vi "Untitled 2 (pub).vi"() -> (0 "error out":errorcluster, 2 "Array 3":dbl[](array[numeric]), 3 "Message":string)   [LabVIEW 2016]
uses:
  builds/UnicornMain/UnicornRIO1/ROS for LabVIEW/home/lvuser/natinst/bin/user.lib/ROS for LabVIEW Software/ROS/Code/SubVIs/_ROSControl.ctl
  builds/UnicornMain/UnicornRIO1/ROS for LabVIEW/home/lvuser/natinst/bin/user.lib/ROS for LabVIEW Software/ROS/Code/SubVIs/_ROSDirection.ctl
  builds/UnicornMain/UnicornRIO1/ROS for LabVIEW/home/lvuser/natinst/bin/user.lib/ROS for LabVIEW Software/ROS/Code/Console/Servers/ServerSubs/TopicDef.ctl
  GlobalVI.vi
  Global 2.vi
  builds/UnicornMain/UnicornRIO1/ROS for LabVIEW/home/lvuser/natinst/bin/user.lib/ROS for LabVIEW Software/ROS/Code/_ROSDefinition.vi
panel:
  out "JSON string 2":string
  out "ROS out":T1={"topic port"=0, "Node"="", "topic"="", "type"="", "node port"=0, "error "={"status"=FALSE, "code"=0, "source"=""}, "Direction"=enum."Node", "Update (ms)"=1, "FIFO size"=1}
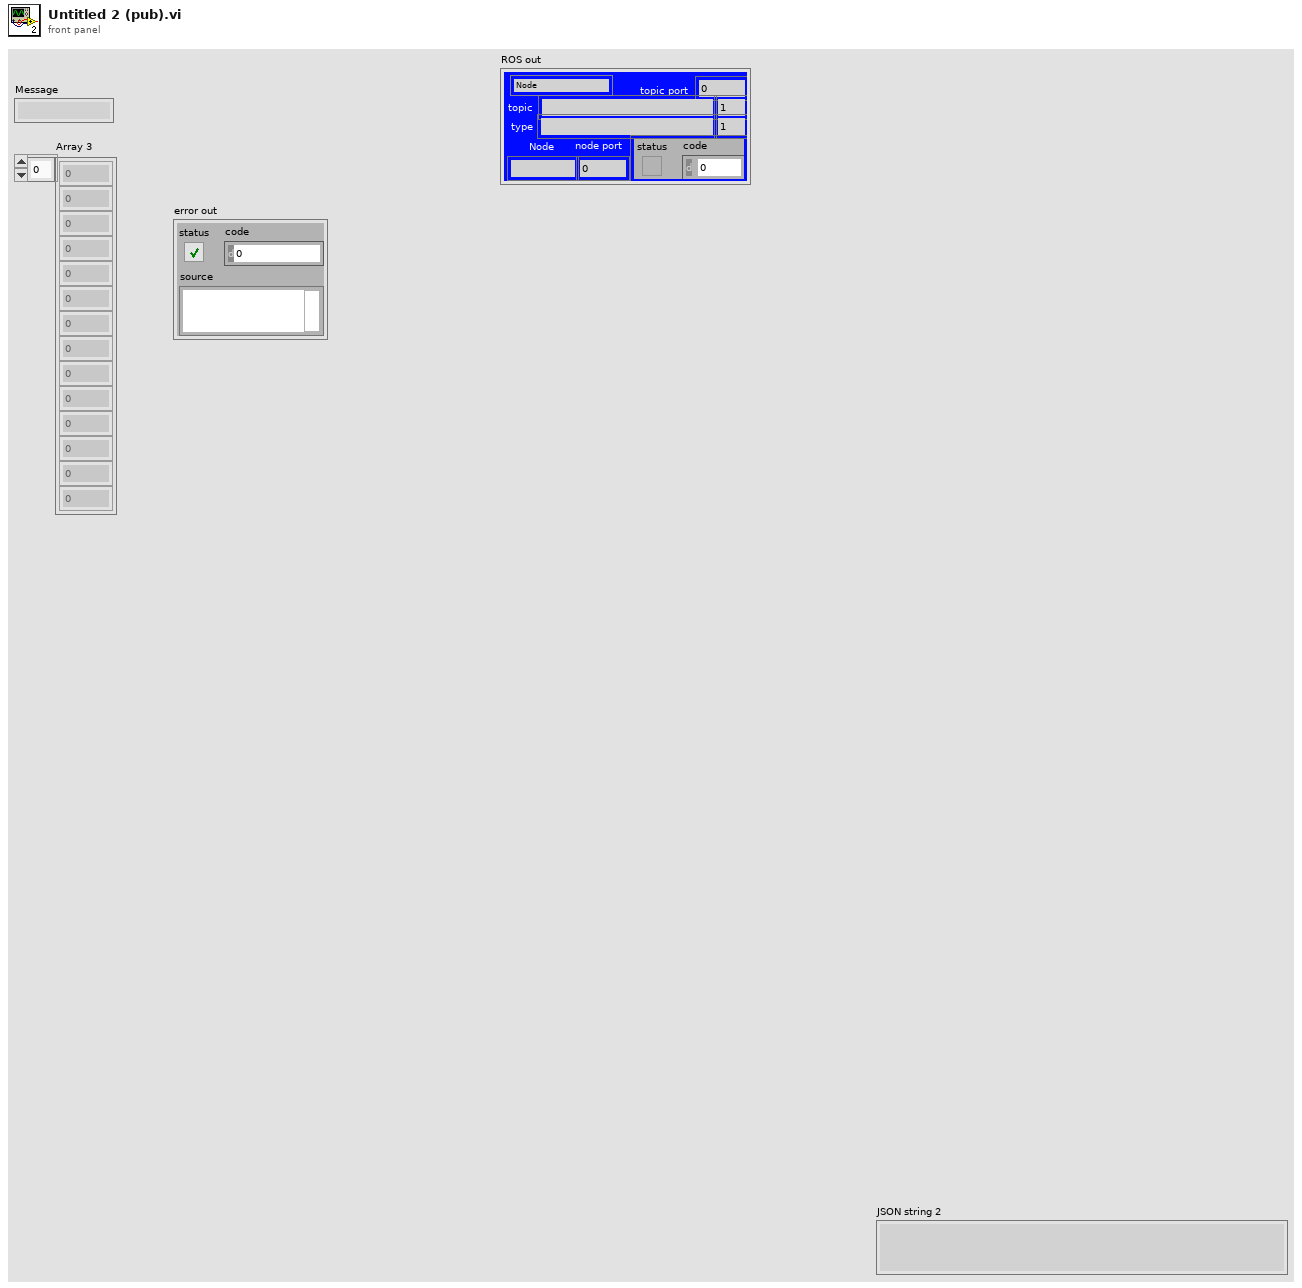
[diagram p1: front panel]
types:
  T1 = typedef "_ROSControl.ctl" = cluster{"topic port":u16, "Node":string, "topic":string, "type":string, "node port":u16, "error ":errorcluster, "Direction":T2, "Update (ms)":u16, "FIFO size":u16}
  T2 = typedef "_ROSDirection.ctl" = enum16{"Node", "Publisher", "Subscriber", "ServiceClient", "ServiceProvider"}
  T3 = typedef "TopicDef.ctl" = cluster{"Topic":string, "Type":string, "Action":T2, "Update (ms)":u16, "queue size":u16}
  T4 = cluster{"status":cluster{"liftStatus":bool, "lidarBackStatus":bool, "uwbStatus":bool, "lightStatus":bool}}
  T5 = cluster{"liftStatus":bool, "lidarBackStatus":bool, "uwbStatus":bool, "lightStatus":bool}
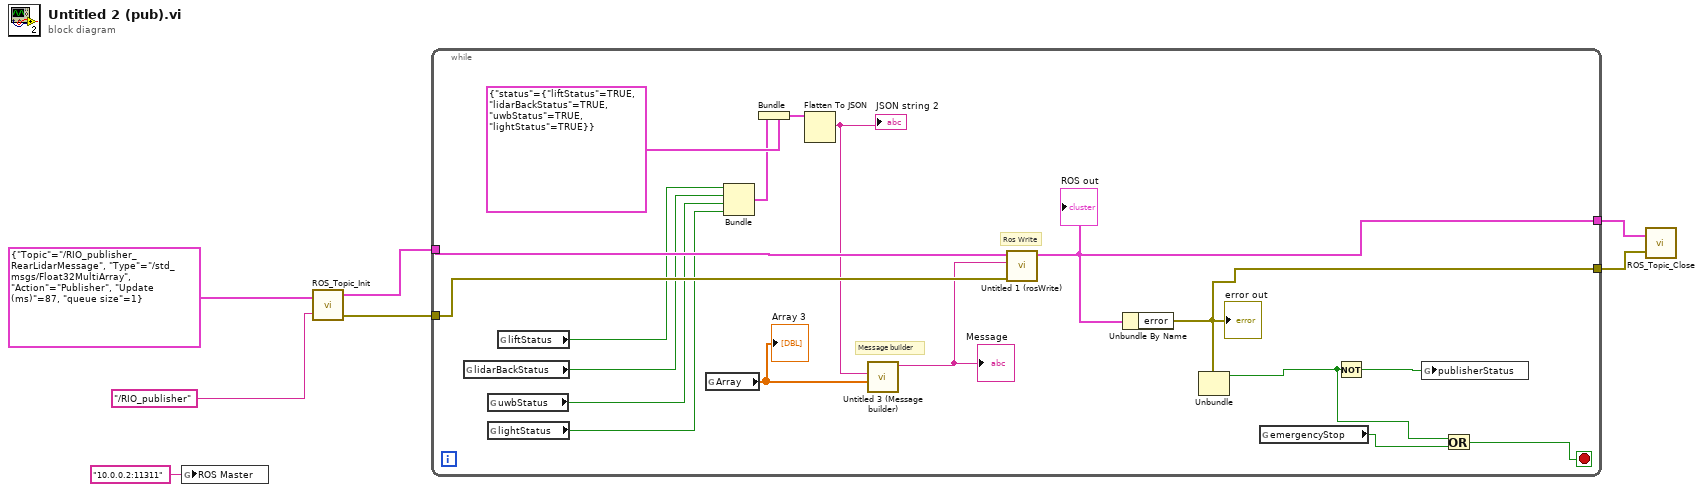
[diagram p0: block diagram]
diagram:
  n1 = global write "_ROSDefinition.vi" "ROS Master"("10.0.0.2:11311" ("ROS Master")) -> ()
  n2 = call "ROS_Topic_Init.vi"("Definitions"=T3 {"Topic"="/RIO_publisher_RearLidarMessage", "Type"="/std_msgs/Float32MultiArray", "Action"=enum."Publisher", "Update (ms)"=87, "queue size"=1}, "node"="/RIO_publisher") -> ("ROS out"=w6:T1, "error out"=w7:errorcluster)  [unwired: 1 in]
  n3 = while {
    tunnel: [w22] -> w4
    tunnel: [w21] -> w5
    tunnel: w6 -> [w19]
    tunnel: w7 -> [w18]
    stop <- w20 stop-if-true
    # "Message builder"
    # "Ros Write"
    n4 = global read "GlobalVI.vi" "lidarBackStatus"() -> (w13:bool)
    n5 = global read "GlobalVI.vi" "uwbStatus"() -> (w12:bool)
    n6 = global read "GlobalVI.vi" "lightStatus"() -> (w11:bool)
    n7 = global read "GlobalVI.vi" "liftStatus"() -> (w14:bool)
    n8 = global read "Global 2.vi" "Array"() -> (w10:dbl[])
    "Array 3" <- w10
    n9 = Bundle("liftStatus"=w14, "lidarBackStatus"=w13, "uwbStatus"=w12, "lightStatus"=w11) -> (w16:T5)  [unwired: 1 in]
    n10 = Bundle(cluster=T4 {"status"={"liftStatus"=TRUE, "lidarBackStatus"=TRUE, "uwbStatus"=TRUE, "lightStatus"=TRUE}}, "status"=w16) -> (w15:T4)
    n11 = Flatten To JSON(anything=w15) -> (JSON string=w8:string)  [unwired: 2 in, 1 out]
    "JSON string 2" <- w8
    n12 = call "Untitled 3 (Message builder).vi"("Array"=w10, "String"=w8) -> ("msg out"=w9:string)  [unwired: 9 in]
    "Message" <- w9
    n13 = call "Untitled 1 (rosWrite).vi"("error in (no error)"=w18, "msg in"=w9, "ROS in"=w19) -> ("ROS out"=w22:T1)  [unwired: 8 in]
    "ROS out" <- w22
    n14 = Unbundle By Name(w22) -> ("error"=w21:errorcluster)
    "error out" <- w21
    n15 = Unbundle(w21) -> ("status"=w23:bool)  [unwired: 2 out]
    n16 = global read "GlobalVI.vi" "emergencyStop"() -> (w24:bool)
    n17 = Not(x=w23) -> (.not. x?=w25:bool)
    n18 = global write "GlobalVI.vi" "publisherStatus"(w25) -> ()
    n19 = Or(x=w23, y=w24) -> (x .or. y?=w20:bool)
  }
  n20 = call "ROS_Topic_Close.vi"("error in"=w5, "ROS in"=w4) -> ()  [unwired: 2 in, 1 out]
